vi "test Add Duplicate Endpoint.vi"(8 "error in (no error)":errorcluster, 11 "TestCase in":refnum<class "Routing and Faulting Aliases Unit Tests.lvclass">) -> (0 "error out":errorcluster, 3 "TestCase out":refnum<class "Routing and Faulting Aliases Unit Tests.lvclass">)   [LabVIEW 2020, in "Routing and Faulting Aliases Unit Tests.lvclass"]
uses:
  Routing and Faulting Aliases Unit Tests.lvclass
  System Explorer/Alias.ctl
  System Explorer/Endpoint.ctl
  Shared/Alias Mapping.ctl
  Shared/Alias Endpoint.ctl
  Routing and Faulting Aliases Unit Tests.lvclass/Routing and Faulting Aliases Unit Tests.ctl
  <vilib>/addons/_JKI Toolkits/VI Tester/TestCase.llb/TestCase.lvclass
  System Explorer/Routing and Faulting System Explorer.lvlib
  Scripting/Routing and Faulting Scripting.lvlib
  Shared/Routing and Faulting Shared.lvlib
  C:/Program Files (x86)/National Instruments/LabVIEW 2020/vi.lib/addons/_JKI Toolkits/VI Tester/TestCase.llb/TestCase.lvclass
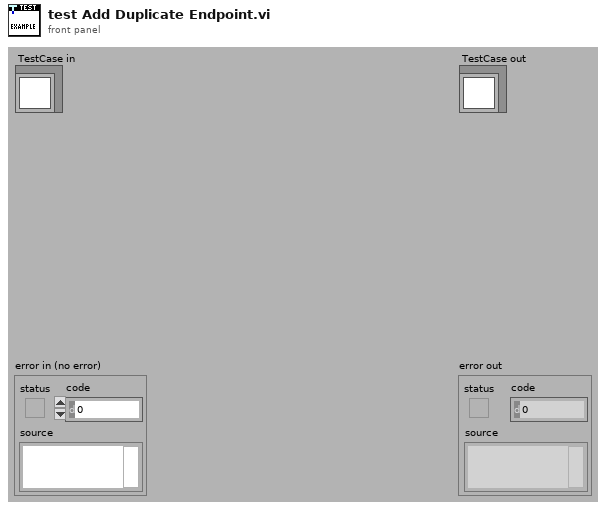
[diagram p1: front panel]
types:
  T1 = typedef "Routing and Faulting Shared.lvlib/Alias Endpoint.ctl" = cluster{"Module Path":string, "Endpoint":string}
  T2 = typedef "Routing and Faulting Shared.lvlib/Alias Mapping.ctl" = cluster{"Alias":string, "Endpoint":T1}
  T3 = typedef "Routing and Faulting System Explorer.lvlib/Endpoint.ctl" = string
  T4 = typedef "Routing and Faulting System Explorer.lvlib/Alias.ctl" = cluster{"Endpoint":T3, "Alias":string, "Remove":bool}
  T5 = typedef "Custom Device API.lvlib/Custom Device Item Ref.ctl" = u64
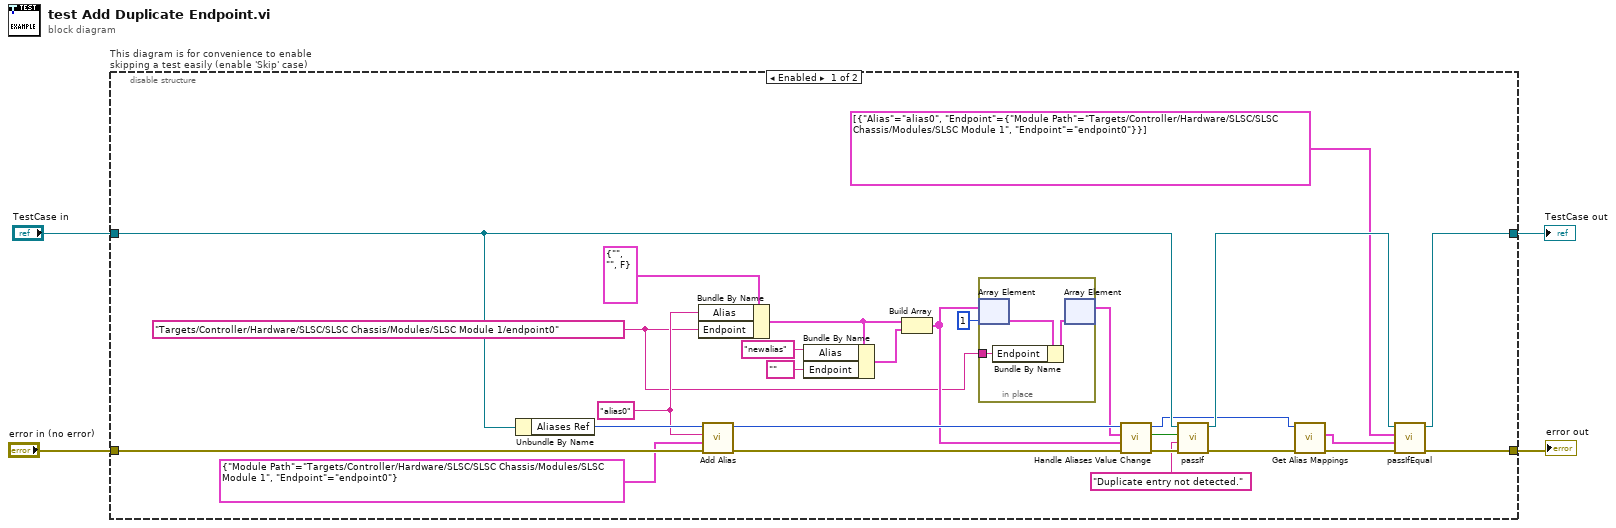
[diagram p0: block diagram]
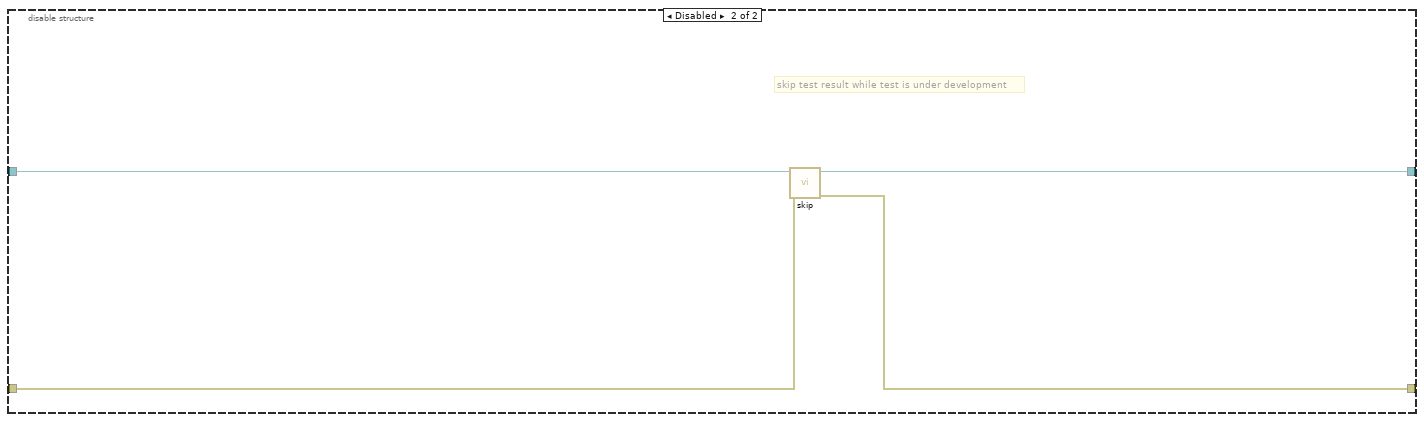
[diagram p2: hidden frame]
diagram:
  n1 = disable-structure "This diagram is for convenience to enable skipping a test easily (enable 'Skip' case)" shown="Enabled" {
    disable-tunnel: "TestCase in" -> [w14 w38]
    disable-tunnel: [w28 w36] -> w1
    disable-tunnel: [w30 w37] -> w3
    disable-tunnel: "error in (no error)" -> [w26 w35]
    frame Enabled {
      w5 = T3 "Targets/Controller/Hardware/SLSC/SLSC Chassis/Modules/SLSC Module 1/endpoint0" ("Endpoint")
      w17 = "alias0" ("Alias")
      n2 = Unbundle By Name(w14) -> ("Aliases Ref"=w27:T5)
      n3 = Bundle By Name(cluster=T4 {"Endpoint"="", "Alias"="", "Remove"=FALSE} ("Alias"), "Alias"=w17, "Endpoint"=w5) -> (w21:T4)
      n4 = call "Add Alias.vi"("error in"=w26, "endpoint"=T1 {"Module Path"="Targets/Controller/Hardware/SLSC/SLSC Chassis/Modules/SLSC Module 1", "Endpoint"="endpoint0"} ("Endpoint"), "alias"=w17, "endpoint aliases in"=w27) -> ("error out"=w24:errorcluster, "endpoint aliases out"=w25:T5)  [unwired: 6 in]
      n5 = Bundle By Name(cluster=w21, "Alias"="newalias", "Endpoint"=T3 "") -> (w20:T4)
      n6 = Build Array(w21, w20) -> (w19:T4[])
      n7 = in-place {
        in-place-border: w5 -> [w32]
        n8 = in-place-array #1(w19, 1) -> (w34:T4)
        n9 = Bundle By Name(cluster=w34, "Endpoint"=w32) -> (w33:T4)
        n10 = in-place-array #1(w33) -> (w16:T4[])  [unwired: 1 out]
      }
      n11 = call "Handle Aliases Value Change.vi"("error in (no error)"=w24, "OldVal"=w19, "NewVal"=w16, "Aliases Ref in"=w25) -> ("error out"=w15:errorcluster, "Duplicate Entry"=w12:bool, "Aliases Ref out"=w9:T5)  [unwired: 4 in, 1 out]
      n12 = call-dynamic "passIf.vi"("error in (no error)"=w15, "message (\"\")"="Duplicate entry not detected." ("message (\"\")"), "pass"=w12, "TestCase in"=w14) -> ("error out"=w10:errorcluster, "TestCase out"=w13:refnum<class "Routing and Faulting Aliases Unit Tests.lvclass">)  [unwired: 6 in]
      n13 = call "Get Alias Mappings.vi"("error in"=w10, "endpoint aliases in"=w9) -> ("error out"=w31:errorcluster, "alias mappings"=w29:T2[])  [unwired: 7 in, 1 out]
      n14 = call-dynamic "passIfEqual.vi"("error in (no error)"=w31, "y"=w29, "x"=T2[] [{"Alias"="alias0", "Endpoint"={"Module Path"="Targets/Controller/Hardware/SLSC/SLSC Chassis/Modules/SLSC Module 1", "Endpoint"="endpoint0"}}] ("Alias Mappings"), "TestCase in"=w13) -> ("error out"=w30:errorcluster, "TestCase out"=w28:refnum<class "Routing and Faulting Aliases Unit Tests.lvclass">)  [unwired: 6 in]
    }
    frame Disabled {
      # "skip test result while test is under development"
      n15 = call <vilib>:"skip.vi"("error in (no error)"=w35, "TestCase in"=w38) -> ("error out"=w37:errorcluster, "TestCase out"=w36:refnum<class "Routing and Faulting Aliases Unit Tests.lvclass">)  [unwired: 8 in]
    }
  }
  "error out" <- w3
  "TestCase out" <- w1
